vi "SRAM Initialized Test.vi"(8 "error in (no error)":errorcluster) -> (0 "error out":errorcluster, 2 "Passed?":string, 3 "Test Result":string)   [LabVIEW 2022 SP3]
uses:
  <vilib>/Instr/_visa.llb/VISA Flush IO Buffer Mask.ctl
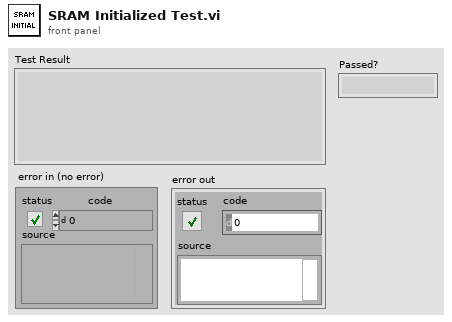
[diagram p1: front panel]
types:
  T1 = typedef "VISA Flush IO Buffer Mask.ctl" = u16
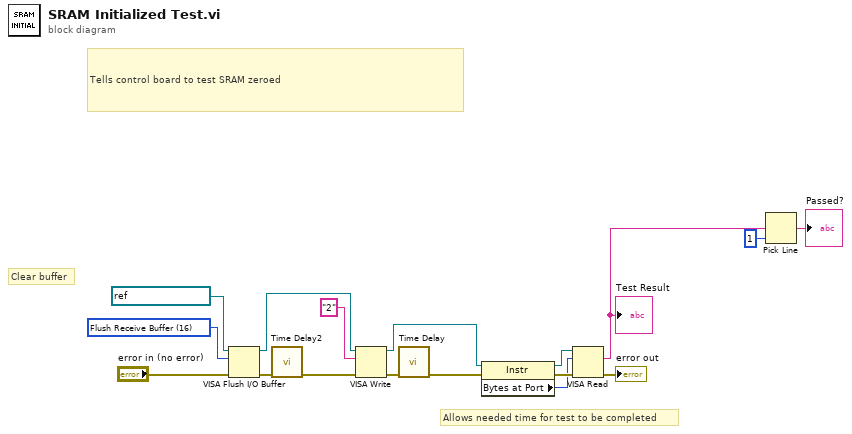
[diagram p0: block diagram]
diagram:
  w16 = T1 16 items=["Flush Receive Buffer"=16, "Write Transmit Buffer to Device"=32, "Flush Receive Buffer (No I/O)"=64, "Flush Transmit Buffer"=128] ("Mask")
  # "Allows needed time for test to be completed"
  # "Tells control board to test SRAM zeroed"
  # "Clear buffer"
  n1 = VISA Flush I/O Buffer(VISA resource name=refnum<visa-resource-name> "ControlBoard", mask (16)=w16, error in (no error)="error in (no error)") -> (VISA resource name out=w14:refnum<visa-resource-name>, error out=w11:errorcluster)
  n2 = call "Time Delay2"("error in (no error)"=w11) -> ("error out"=w10:errorcluster)  [unwired: 10 in]
  n3 = VISA Write(VISA resource name=w14, write buffer="2", error in (no error)=w10) -> (VISA resource name out=w8:refnum<visa-resource-name>, error out=w15:errorcluster)  [unwired: 1 out]
  n4 = call "Time Delay"("error in (no error)"=w15) -> ("error out"=w9:errorcluster)  [unwired: 10 in]
  n5 = property class="Instr"(reference=w8, error in=w9) -> (reference out=w7:refnum<visa-resource-name>, error out=w6:errorcluster, "Bytes at Port"=w5:u32)
  n6 = VISA Read(VISA resource name=w7, byte count=w5, error in (no error)=w6) -> (read buffer=w3:string, error out=→"error out":errorcluster)  [unwired: 2 out]
  "Test Result" <- w3
  n7 = Pick Line(multi-line string=w3, line index=1) -> (output string=→"Passed?":string)  [unwired: 1 in]
